vi "sub_device1.vi"   [LabVIEW 2017]
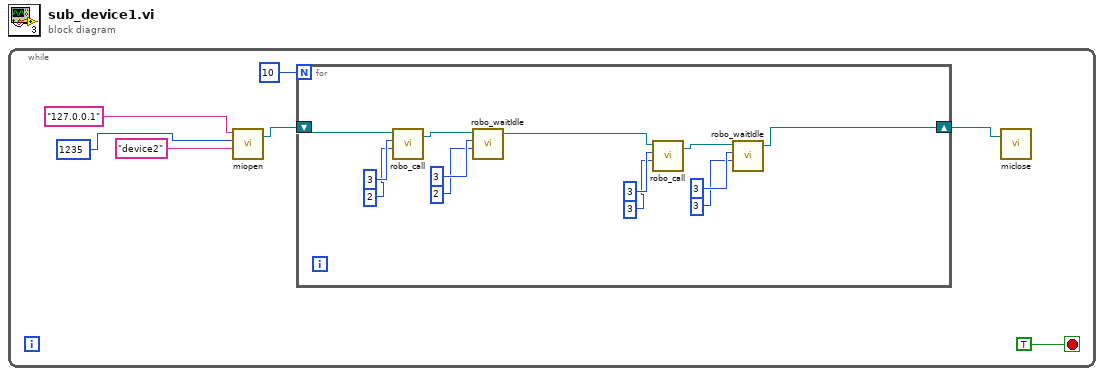
[diagram p0: block diagram]
diagram:
  n1 = while {
    stop <- TRUE stop-if-true
    n2 = call "miopen.vi"("name"="device2", "port"=u16 1235, "ip"="127.0.0.1") -> ("VISA资源名称输出"=w3:refnum<visa-resource-name>)  [unwired: 1 in, 1 out]
    n3 = for {
      N: 10 -> [_]
      shift-right: [w8] -> w7
      shift-left: w3 -> [w15]
      n4 = call "robo_call.vi"("page"=2, "ax"=3, "VISA资源名称"=w15) -> ("VISA资源名称输出"=w16:refnum<visa-resource-name>)  [unwired: 3 in, 1 out]
      n5 = call "robo_waitIdle.vi"("VISA资源名称"=w16, "ax"=3, "page"=2) -> ("VISA资源名称输出"=w9:refnum<visa-resource-name>)  [unwired: 2 in, 2 out]
      n6 = call "robo_call.vi"("page"=3, "ax"=3, "VISA资源名称"=w9) -> ("VISA资源名称输出"=w10:refnum<visa-resource-name>)  [unwired: 3 in, 1 out]
      n7 = call "robo_waitIdle.vi"("VISA资源名称"=w10, "ax"=3, "page"=3) -> ("VISA资源名称输出"=w8:refnum<visa-resource-name>)  [unwired: 2 in, 2 out]
    }
    n8 = call "miclose.vi"("VISA资源名称"=w7) -> ()  [unwired: 1 in, 1 out]
  }
